vi "ScriptClass.vi"(0 "reference in":refnum<class "Executer.lvclass">, 1 "Path":path, 2 "Name":string, 3 "Scripting":refnum<class "Scripting.lvclass">, 5 "error in (no error)":errorcluster) -> (14 "reference out":refnum<class "Executer.lvclass">, 19 "error out":errorcluster)   [LabVIEW 2018, in "Executer.lvclass"]
uses:
  Executer.lvclass
  Scripting/Scripting_class/Scripting.lvclass
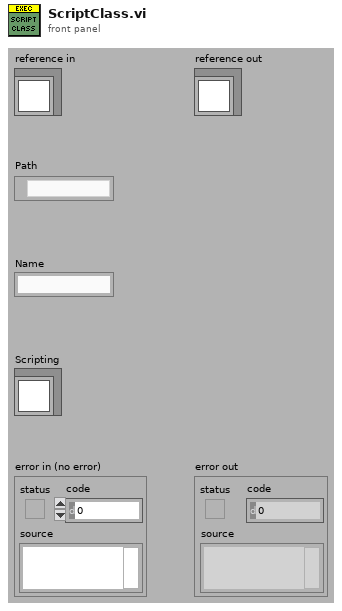
[diagram p1: front panel]
types:
  T1 = typedef "Executer.lvclass/ClassDescription.ctl" = cluster{"ClassName":string, "ClassDescription":string, "MethodDescriptions":T2[]}
  T2 = typedef "Executer.lvclass/MethodDescription.ctl" = cluster{"MethodName":string, "VIDescription":string, "ControlDesciptions":string[], "IndicatorDesciptions":string[], "ControlTypes":variant[], "IndicatorTypes":variant[]}
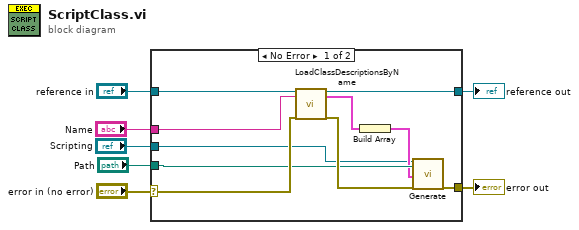
[diagram p0: block diagram]
diagram:
  n1 = case shown="No Error" "error in (no error)" {
    selector: "error in (no error)" -> [w16 w19]
    tunnel: [w17 w19] -> w6
    tunnel: [w14 w18] -> w4
    tunnel: "reference in" -> [w15 w18]
    tunnel: "Name" -> [w12 _]
    tunnel: "Path" -> [w11 _]
    tunnel: "Scripting" -> [w8 _]
    frame No Error {
      n2 = call "LoadClassDescriptionsByName.vi"("Executer in"=w15, "Class in"=w12, "error in (no error)"=w16) -> ("Executer out"=w14:refnum<class "Executer.lvclass">, "ClassDescription"=w10:T1, "error out"=w13:errorcluster)  [unwired: 14 in]
      n3 = Build Array(w10) -> (w9:T1[])
      n4 = call-dynamic "Generate.vi"("reference in"=w8, "Path"=w11, "Classes"=w9, "error in (no error)"=w13) -> ("error out"=w17:errorcluster)  [unwired: 14 in, 1 out]
    }
    frame Error {
    }
  }
  "error out" <- w6
  "reference out" <- w4
